vi "P30_Count2.vi"() -> ()   [LabVIEW 2022 SP3]
panel:
  out "a 2":bool
  out "g 2":bool
  out "d 2":bool
  out "b 2":bool
  out "c 2":bool
  out "f 2":bool
  out "e 2":bool
  in  "Reset":bool
  in  "Start/Pause":bool
  in  "Stop":bool
  in  "T":bool
  out "a":bool
  out "g":bool
  out "d":bool
  out "b":bool
  out "c":bool
  out "f":bool
  out "e":bool
  out "Numeric":u32
  in  "s/p":bool
  in  "Up":bool
  # "P30_Count2"
  # "Equipo C\nJairo Issac García López\nRodolfo Durón Hernandez\nRoberto Carlos Herrera Pérez\nSebastián Rodríguez Posada"
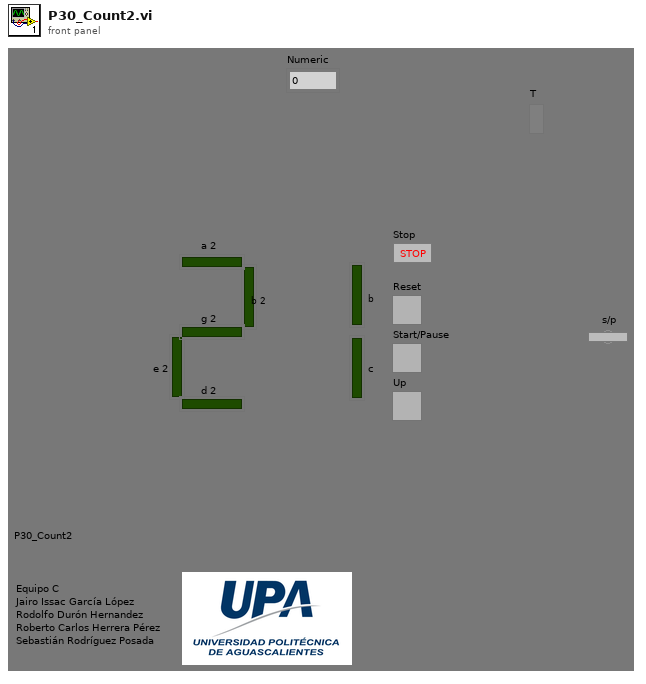
[diagram p1: front panel]
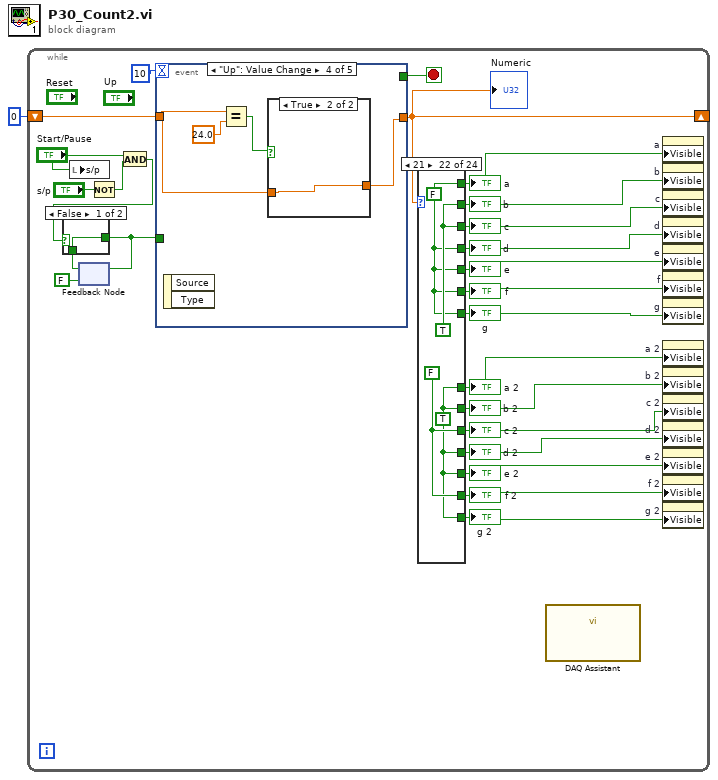
[diagram p0: block diagram]
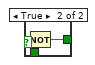
[diagram p2: hidden frame]
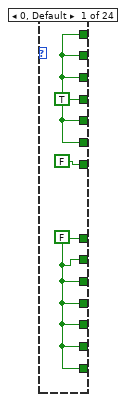
[diagram p3: hidden frame]
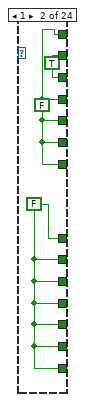
[diagram p4: hidden frame]
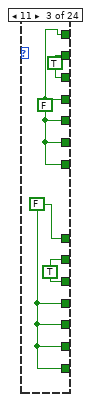
[diagram p5: hidden frame]
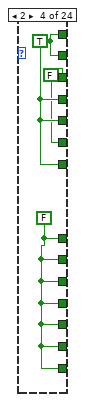
[diagram p6: hidden frame]
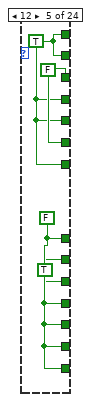
[diagram p7: hidden frame]
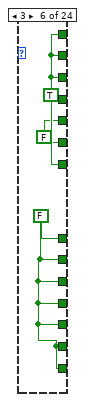
[diagram p8: hidden frame]
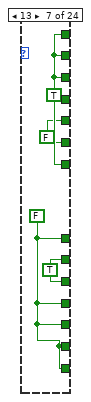
[diagram p9: hidden frame]
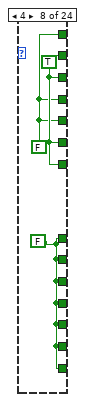
[diagram p10: hidden frame]
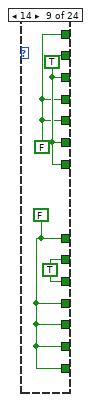
[diagram p11: hidden frame]
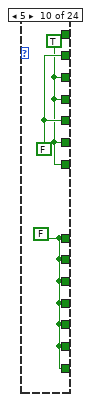
[diagram p12: hidden frame]
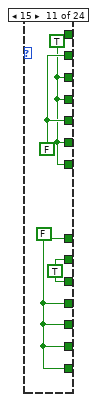
[diagram p13: hidden frame]
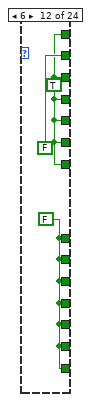
[diagram p14: hidden frame]
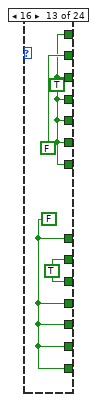
[diagram p15: hidden frame]
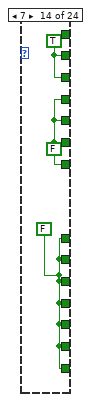
[diagram p16: hidden frame]
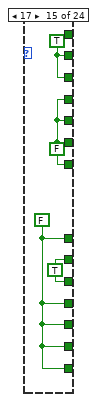
[diagram p17: hidden frame]
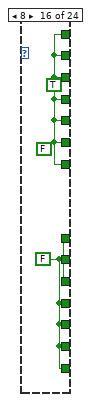
[diagram p18: hidden frame]
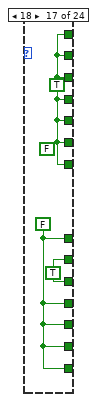
[diagram p19: hidden frame]
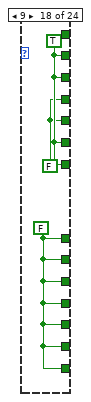
[diagram p20: hidden frame]
diagram:
  n1 = while {
    shift-right: [w15] -> _
    shift-left: u16 0 -> [w26]
    stop <- w14 stop-if-true
    n2 = local write "s/p"("Start/Pause") -> ()
    n3 = feedback #1(FALSE) -> (w17:bool)
    n4 = Not(x="s/p") -> (.not. x?=w20:bool)
    n5 = And(x="Start/Pause", y=w20) -> (x .and. y?=w19:bool)
    n6 = case shown="False" w19 {
      tunnel: [w27 w29] -> w18
      tunnel: w17 -> [w27 w28]
      frame False {
      }
      frame True {
        n7 = Not(x=w28) -> (.not. x?=w29:bool)
      }
    }
    n8 = feedback-in #1(w18) -> ()
    n9 = event shown="[3] \"Up\": Value Change" {
      selector: _ -> [_ _ _ _ _]
      dyn-events: _ -> [_ _ _ _ _]
      timeout: 10 -> [_ _ _ _ _]
      tunnel: w26 -> [w119 w130 _ w133 _]
      tunnel: [w116 w131 _ w134 0] -> w15
      tunnel: w18 -> [w114 _ _ _ _]
      tunnel: [_ _ "Stop" _ _] -> w14
      event Timeout {
        n10 = event-data() -> ()  [unwired: 1 in, 1 out]
        n11 = case shown="True" w114 {
          tunnel: w119 -> [w122 w124]
          tunnel: [w122 w123] -> w115
          frame False {
          }
          frame True {
            w125 = 0.25
            n12 = flat-sequence {
              tunnel: w125 -> [w126]
              tunnel: w125 -> [w128]
              frame #0 {
                n13 = call "D"("Delay Time (s)"=w126) -> ()  [unwired: 10 in, 1 out]
                n14 = local write "T"(TRUE) -> ()
              }
              frame #1 {
                n15 = call "D2"("Delay Time (s)"=w128) -> ()  [unwired: 10 in, 1 out]
                n16 = local write "T"(FALSE) -> ()
              }
            }
            n17 = Increment(x=w124) -> (x+1=w123:dbl)
          }
        }
        n18 = Equal?(x=w115, y=24) -> (x = y?=w118:bool)
        n19 = case shown="True" w118 {
          tunnel: [w120 0] -> w116
          tunnel: w115 -> [w120 _]
          frame False {
          }
          frame True {
          }
        }
      }
      event "T": Value Change {
        n20 = event-data() -> ()  [unwired: 1 in, 3 out]
        n21 = Increment(x=w130) -> (x+1=w131:dbl)
      }
      event "Stop": Value Change {
        n22 = event-data() -> ()  [unwired: 1 in, 3 out]
      }
      event "Up": Value Change {
        n23 = event-data() -> ()  [unwired: 1 in, 2 out]
        n24 = Equal?(x=w133, y=24.0) -> (x = y?=w135:bool)
        n25 = case shown="True" w135 {
          tunnel: [w139 w140] -> w134
          tunnel: w133 -> [w137 w140]
          frame False {
            n26 = Add(x=0.5, y=w137) -> (x+y=w139:dbl)
          }
          frame True {
          }
        }
      }
      event "Reset": Value Change {
        n27 = event-data() -> ()  [unwired: 1 in, 6 out]
      }
    }
    "Numeric" <- w15
    n28 = case shown="21" w15 {
      tunnel: [w32 w34 w38 w42 w44 w49 w53 w55 w59 w62 w66 w69 w73 w77 w81 w83 w86 w89 w93 w95 w101 w102 w107 w111] -> w24
      tunnel: [w32 w34 w38 w41 w46 w48 w52 w56 w60 w62 w66 w69 w73 w76 w80 w83 w86 w89 w93 w95 w101 w102 w106 w110] -> w23
      tunnel: [w30 w33 w37 w40 w45 w47 w51 w54 w58 w61 w65 w68 w72 w75 w79 w82 w85 w87 w91 w97 w99 w105 w109 w113] -> w13
      tunnel: [w30 w33 w36 w40 w43 w47 w50 w54 w57 w61 w64 w68 w71 w75 w78 w82 w84 w87 w90 w96 w98 w104 w108 w112] -> w12
      tunnel: [w30 w33 w37 w40 w45 w47 w51 w54 w58 w61 w65 w68 w72 w75 w79 w82 w85 w87 w91 w97 w98 w104 w108 w112] -> w11
      tunnel: [w30 w33 w37 w40 w45 w47 w51 w54 w58 w61 w65 w68 w72 w75 w79 w82 w85 w87 w91 w97 w98 w104 w108 w112] -> w10
      tunnel: [w30 w33 w37 w40 w45 w47 w51 w54 w58 w61 w65 w68 w72 w75 w79 w82 w85 w87 w91 w97 w98 w104 w108 w112] -> w9
      tunnel: [w30 w33 w36 w40 w43 w47 w50 w54 w57 w61 w64 w68 w71 w75 w78 w82 w84 w87 w90 w96 w99 w105 w109 w113] -> w8
      tunnel: [w30 w33 w37 w40 w45 w47 w51 w54 w58 w61 w65 w68 w72 w75 w79 w82 w85 w87 w91 w97 w98 w104 w108 w112] -> w7
      tunnel: [w32 w35 w39 w42 w44 w49 w53 w56 w60 w63 w67 FALSE FALSE w77 w81 w83 w86 w89 w93 w95 w101 w103 w107 w111] -> w6
      tunnel: [w32 w35 w39 w41 w46 w49 w53 w56 w60 w62 w66 w69 w73 w77 w81 w83 w86 w89 w93 w95 w101 w103 w106 w111] -> w5
      tunnel: [w32 w34 w38 w42 w44 w49 w53 w55 w59 w62 w66 w69 w73 w76 w80 w83 w86 w88 w92 w95 w101 w102 w107 w111] -> w4
      tunnel: [w32 w34 w38 w42 w44 w48 w52 w55 w59 w63 w67 w69 w73 w76 w80 w83 w86 w88 w92 w95 w101 w102 w107 w110] -> w3
      tunnel: [FALSE w34 w38 w42 w44 w49 w53 w56 w60 w62 w66 w69 w73 w76 w80 w83 w86 w89 w93 FALSE FALSE w102 w107 w111] -> w2
      frame 0, Default {
        w30 = FALSE
        w32 = TRUE
      }
      frame 1 {
        w33 = FALSE
        w34 = FALSE
        w35 = TRUE
      }
      frame 11 {
        w36 = TRUE
        w37 = FALSE
        w38 = FALSE
        w39 = TRUE
      }
      frame 2 {
        w40 = FALSE
        w41 = FALSE
        w42 = TRUE
      }
      frame 12 {
        w43 = TRUE
        w45 = FALSE
        w46 = FALSE
        w44 = TRUE
      }
      frame 3 {
        w47 = FALSE
        w48 = FALSE
        w49 = TRUE
      }
      frame 13 {
        w50 = TRUE
        w51 = FALSE
        w52 = FALSE
        w53 = TRUE
      }
      frame 4 {
        w54 = FALSE
        w55 = FALSE
        w56 = TRUE
      }
      frame 14 {
        w57 = TRUE
        w58 = FALSE
        w59 = FALSE
        w60 = TRUE
      }
      frame 5 {
        w61 = FALSE
        w63 = FALSE
        w62 = TRUE
      }
      frame 15 {
        w64 = TRUE
        w65 = FALSE
        w67 = FALSE
        w66 = TRUE
      }
      frame 6 {
        w68 = FALSE
        w69 = TRUE
      }
      frame 16 {
        w71 = TRUE
        w72 = FALSE
        w73 = TRUE
      }
      frame 7 {
        w75 = FALSE
        w76 = FALSE
        w77 = TRUE
      }
      frame 17 {
        w78 = TRUE
        w79 = FALSE
        w80 = FALSE
        w81 = TRUE
      }
      frame 8 {
        w82 = FALSE
        (unwired) FALSE
        w83 = TRUE
      }
      frame 18 {
        w84 = TRUE
        w85 = FALSE
        (unwired) FALSE
        w86 = TRUE
      }
      frame 9 {
        w87 = FALSE
        w88 = FALSE
        w89 = TRUE
      }
      frame 19 {
        w90 = TRUE
        w91 = FALSE
        w92 = FALSE
        w93 = TRUE
      }
      frame 10 {
        w96 = TRUE
        w97 = FALSE
        w95 = TRUE
      }
      frame 20 {
        w98 = TRUE
        w99 = FALSE
        w101 = TRUE
      }
      frame 21 {
        w103 = TRUE
        w104 = TRUE
        w105 = FALSE
        w102 = FALSE
      }
      frame 22 {
        w106 = FALSE
        w108 = TRUE
        w109 = FALSE
        w107 = TRUE
      }
      frame 23 {
        w110 = FALSE
        w112 = TRUE
        w113 = FALSE
        w111 = TRUE
      }
    }
    "a" <- w24
    "g" <- w2
    "d" <- w4
    "b" <- w6
    "c" <- w5
    "f" <- w23
    "e" <- w3
    "a 2" <- w11
    "g 2" <- w7
    "d 2" <- w10
    "b 2" <- w12
    "c 2" <- w8
    "f 2" <- w13
    "e 2" <- w9
    n29 = call "DAQ Assistant"() -> ()  [unwired: 12 in]
    n30 = property on="a" class="Bool (strict)"("Visible"=w24) -> ()  [unwired: 2 in, 2 out]
    n31 = property on="b" class="Bool (strict)"("Visible"=w6) -> ()  [unwired: 2 in, 2 out]
    n32 = property on="c" class="Bool (strict)"("Visible"=w5) -> ()  [unwired: 2 in, 2 out]
    n33 = property on="d" class="Bool (strict)"("Visible"=w4) -> ()  [unwired: 2 in, 2 out]
    n34 = property on="e" class="Bool (strict)"("Visible"=w3) -> ()  [unwired: 2 in, 2 out]
    n35 = property on="f" class="Bool (strict)"("Visible"=w23) -> ()  [unwired: 2 in, 2 out]
    n36 = property on="g" class="Bool (strict)"("Visible"=w2) -> ()  [unwired: 2 in, 2 out]
    n37 = property on="a 2" class="Bool (strict)"("Visible"=w11) -> ()  [unwired: 2 in, 2 out]
    n38 = property on="b 2" class="Bool (strict)"("Visible"=w12) -> ()  [unwired: 2 in, 2 out]
    n39 = property on="c 2" class="Bool (strict)"("Visible"=w8) -> ()  [unwired: 2 in, 2 out]
    n40 = property on="d 2" class="Bool (strict)"("Visible"=w10) -> ()  [unwired: 2 in, 2 out]
    n41 = property on="e 2" class="Bool (strict)"("Visible"=w9) -> ()  [unwired: 2 in, 2 out]
    n42 = property on="f 2" class="Bool (strict)"("Visible"=w13) -> ()  [unwired: 2 in, 2 out]
    n43 = property on="g 2" class="Bool (strict)"("Visible"=w7) -> ()  [unwired: 2 in, 2 out]
  }
